vi "Score Particles.vi"(8 "Area Size Limit":i32=444, 9 "Particle Count Limit":i32=10, 11 "Image Refnum in":T1) -> (2 "Scored Particle Info":T2(array[cluster]), 3 "Image Refnum out":T1)   [LabVIEW 2012]
doc: "Score the largest particles in the image to determine how well they match the target attributes. Specifically, calculate how rectangular a particle is, inspect its aspect ratio, and determine if it is hollow (having pixels on around the edges, but off in the large center)."
uses:
  <vilib>/vision/Image Controls.llb/IMAQ Image.ctl
  <vilib>/vision/NI_Vision_Development_Module.lvlib
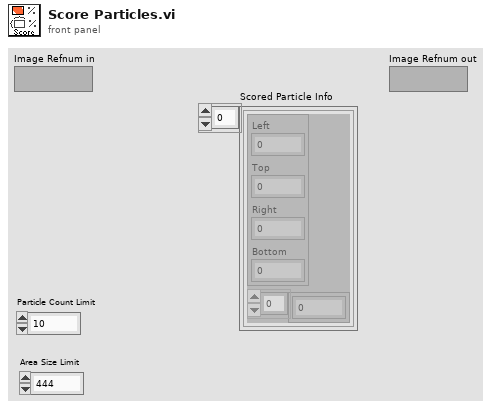
[diagram p1: front panel]
types:
  T1 = typedef "IMAQ Image.ctl" = refnum<image>
  T2 = cluster{cluster{"Left":dbl, "Top":dbl, "Right":dbl, "Bottom":dbl}, dbl[]}[]
  T3 = typedef "Particle Parameters" = i32
  T4 = typedef "Image Type" = u32
  T5 = cluster{"Left":dbl, "Top":dbl, "Right":dbl, "Bottom":dbl}
  T6 = cluster{cluster{"Left":dbl, "Top":dbl, "Right":dbl, "Bottom":dbl}, dbl[]}
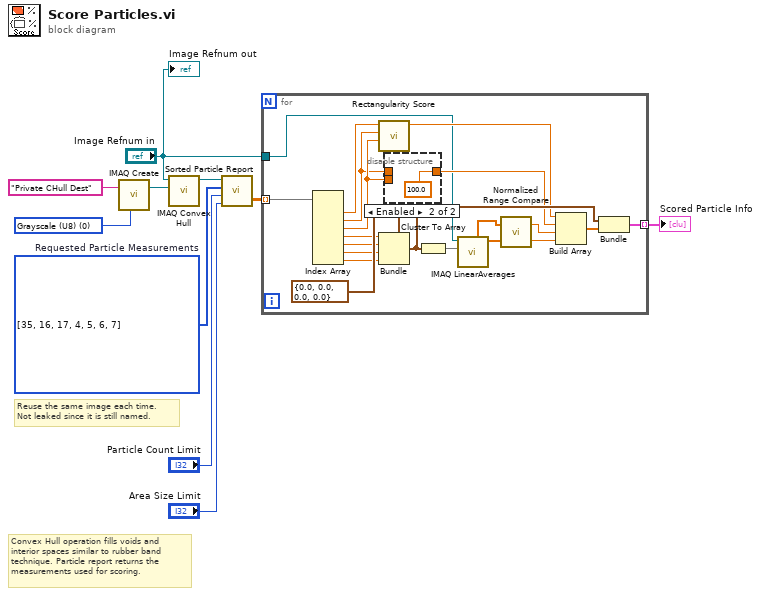
[diagram p0: block diagram]
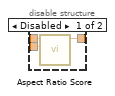
[diagram p2: hidden frame]
diagram:
  w1 = T3[] [35, 16, 17, 4, 5, 6, 7] items=["Center of Mass X", "Center of Mass Y", "First Pixel X", "First Pixel Y", "Bounding Rect Left", "Bounding Rect Top", "Bounding Rect Right", "Bounding Rect Bottom", "Max Feret Diameter Start X", "Max Feret Diameter Start Y", "Max Feret Diameter End X", "Max Feret Diameter End Y", "Max Horiz. Segment Length Left", "Max Horiz. Segment Length Right", "Max Horiz. Segment Length Row", "-", "Bounding Rect Width", "Bounding Rect Height", "Bounding Rect Diagonal", "Perimeter", "Convex Hull Perimeter", "Holes' Perimeter", "Max Feret Diameter", "Equivalent Ellipse Major Axis", "Equivalent Ellipse Minor Axis", "Equivalent Ellipse Minor Axis (Feret)", "Equivalent Rect Long Side", "Equivalent Rect Short Side", "Equivalent Rect Diagonal", "Equivalent Rect Short Side (Feret)", "Average Horiz. Segment Length", "Average Vert. Segment Length", "Hydraulic Radius", "Waddel Disk Diameter", "-", "Area", "Holes' Area", "Particle & Holes' Area", "Convex Hull Area", "Image Area", "-", "Number of Holes", "Number of Horiz. Segments", "Number of Vert. Segments", "-", "Orientation", "Max Feret Diameter Orientation", "-", "% Area/Image Area", "% Area/(Particle & Holes' Area)", "Ratio of Equivalent Ellipse Axes", "Ratio of Equivalent Rect Sides", "-", "Elongation Factor", "Compactness Factor", "Heywood Circularity Factor", "Type Factor", "-", "Sum X", "Sum Y", "Sum XX", "Sum XY", "Sum YY", "Sum XXX", "Sum XXY", "Sum XYY", "Sum YYY", "-", "Moment of Inertia XX", "Moment of Inertia XY", "Moment of Inertia YY", "Moment of Inertia XXX", "Moment of Inertia XXY", "Moment of Inertia XYY", "Moment of Inertia YYY", "Norm. Moment of Inertia XX", "Norm. Moment of Inertia XY", "Norm. Moment of Inertia YY", "Norm. Moment of Inertia XXX", "Norm. Moment of Inertia XXY", "Norm. Moment of Inertia XYY", "Norm. Moment of Inertia YYY", "Hu Moment 1", "Hu Moment 2", "Hu Moment 3", "Hu Moment 4", "Hu Moment 5", "Hu Moment 6", "Hu Moment 7"]  # Requested Particle Measurements
  w7 = T4 0 items=["Grayscale (U8)", "Grayscale (I16)", "Grayscale (SGL)", "Complex (CSG)", "RGB (U32)", "HSL (U32)", "RGB (U64)", "Grayscale (U16)"] ("Image Type")
  # "Reuse the same image each time.\nNot leaked since it is still named."
  # "Convex Hull operation fills voids and\ninterior spaces similar to rubber band\ntechnique. Particle report returns the\nmeasurements used for scoring."
  n1 = call "IMAQ Create"("Image Name"="Private CHull Dest", "Image Type"=w7) -> ("New Image"=w6:T1)  [unwired: 2 in, 2 out]
  n2 = call "IMAQ Convex Hull"("Image Dst"=w6, "Image Src"="Image Refnum in") -> ("Image Dst Out"=w4:T1)  [unwired: 2 in, 7 out]
  n3 = call "Sorted Particle Report.vi"("Area Size Limit"="Area Size Limit", "Particle Count Limit"="Particle Count Limit", "Pixel Measurements"=w1, "Image in"=w4) -> ("Sorted Data"=w9:dbl[][])  [unwired: 1 out]
  n4 = for {
    tunnel: [w28] -> w10 mode=indexing
    tunnel: "Image Refnum in" -> [w18]
    tunnel: w9 -> [w17] mode=indexing
    n5 = Index Array(array=w17) -> (element #1=w29:dbl, element #2=w11:dbl, element #3=w12:dbl, element #4=w13:dbl, element #5=w14:dbl, element #6=w15:dbl, element #7=w16:dbl)  [unwired: 7 in]
    n6 = call "Rectangularity Score.vi"("Height"=w12, "Width"=w11, "Area"=w29) -> ("Score"=w22:dbl)  [unwired: 8 in]
    n7 = Bundle(cluster=T5 {"Left"=0.0, "Top"=0.0, "Right"=0.0, "Bottom"=0.0}, "Left"=w13, "Top"=w14, "Right"=w15, "Bottom"=w16) -> (w27:T5)
    n8 = disable-structure shown="Enabled" {
      disable-tunnel: [w33 100.0] -> w23
      disable-tunnel: w12 -> [w32 _]
      disable-tunnel: w11 -> [w31 _]
      frame Disabled {
        n9 = call "Aspect Ratio Score.vi"("Height"=w32, "Width"=w31) -> ("Score"=w33:dbl)  [unwired: 9 in]
      }
      frame Enabled {
      }
    }
    n10 = Cluster To Array(cluster=w27) -> (array=w19:dbl[])
    n11 = call "IMAQ LinearAverages"("Optional Rectangle"=w19, "Image Src"=w18) -> ("Y Axis Averages"=w21:sgl[], "X Axis Averages"=w20:sgl[])  [unwired: 2 in, 6 out]
    n12 = call "Normalized Range Compare.vi"("Y Averages"=w21, "X Averages"=w20) -> ("Y Score"=w25:dbl, "X Score"=w24:dbl)
    n13 = Build Array(w22, w23, w24, w25) -> (w26:dbl[])
    n14 = Bundle(w27, w26) -> (w28:T6)  [unwired: 1 in]
  }
  "Scored Particle Info" <- w10
  "Image Refnum out" <- "Image Refnum in"
